vi "ma_Generate Multitone Phases.vi"(1 "phase relationship":u16(ring) items=["random", "linear difference", "linear phase"], 2 "seed":i32=-1, 3 "#tones":i32=10) -> (0 "Tone Phases":dbl[](array[numeric]) format="%0.2f")   [LabVIEW 2020, in "NI_MAPro.lvlib"]
uses:
  NI_MAPro.lvlib
  NI_AALBase.lvlib
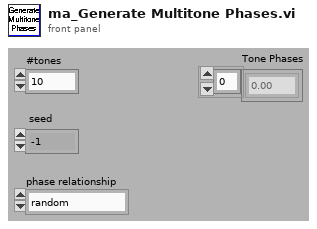
[diagram p1: front panel]
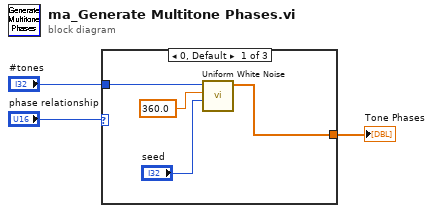
[diagram p0: block diagram]
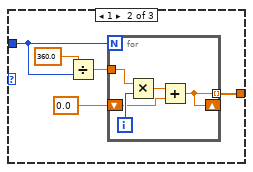
[diagram p2: hidden frame]
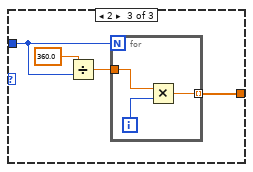
[diagram p3: hidden frame]
diagram:
  n1 = case shown="0, Default" "phase relationship" {
    tunnel: "#tones" -> [w7 w9 w19]
    tunnel: [w4 w10 w20] -> w3
    frame 0, Default {
      n2 = call "Uniform White Noise.vi"("seed"="seed", "amplitude"=360.0 ("y"), "samples"=w7) -> ("uniform white noise"=w4:dbl[])  [unwired: 7 in, 1 out]
    }
    frame 1 {
      n3 = Divide(x=360.0, y=w9) -> (x/y=w12:dbl)
      n4 = for {
        N: w9 -> [_]
        tunnel: w12 -> [w17]
        shift-right: [w13] -> _
        shift-left: 0.0 -> [w14]
        tunnel: [w13] -> w10 mode=indexing
        i -> [w16]
        n5 = Multiply(x=w17, y=w16) -> (x*y=w15:dbl)
        n6 = Add(x=w15, y=w14) -> (x+y=w13:dbl)
      }
    }
    frame 2 {
      n7 = Divide(x=360.0, y=w19) -> (x/y=w21:dbl)
      n8 = for {
        N: w19 -> [_]
        tunnel: w21 -> [w24]
        tunnel: [w22] -> w20 mode=indexing
        i -> [w23]
        n9 = Multiply(x=w24, y=w23) -> (x*y=w22:dbl)
      }
    }
  }
  "Tone Phases" <- w3
